vi "纳清蓝绿藻电极校准.vi"() -> ()   [LabVIEW 2016, in "斯坦道多参数.lvlib"]
uses:
  <vilib>/Utility/miscctls.llb/LVPointTypeDef.ctl
  <vilib>/Utility/miscctls.llb/LVPositionTypeDef.ctl
  <vilib>/Analysis/NI_AALBase.lvlib
panel:
  out "报警信息":string
  out "通讯状态":string
  out "温度校准参数":sgl
  out "第三点校准值":dbl
  out "标液3":sgl
  out "第二点校准值":dbl
  out "第一点校准值":dbl
  in  "校准停止":bool
  in  "校准启动":bool
  in  "校准模式":enum16{"两点校准", "单点校准", "三点校准"}(ring)=enum."单点校准"
  out "最小值":sgl format="%#.2f"
  out "最大值":sgl format="%#.2f"
  out "波形图表":u16(graph) caption="历史曲线"
  out "mean":dbl caption="均值" format="%#.2f"
  out "standard deviation":dbl caption="标准差" format="%#.2f"
  out "变异系数":dbl format="%#.6f"
  out "测量值":sgl
  out "提示":string
  out "标液2":sgl
  out "标液1":sgl
  out "原始光强数值":u16 caption="信号值"
  out "温度":dbl
  # "藻密度电极设定"
  # "℃"
  # "ug/L"
  # "℃"
  # "请选择校准模式:"
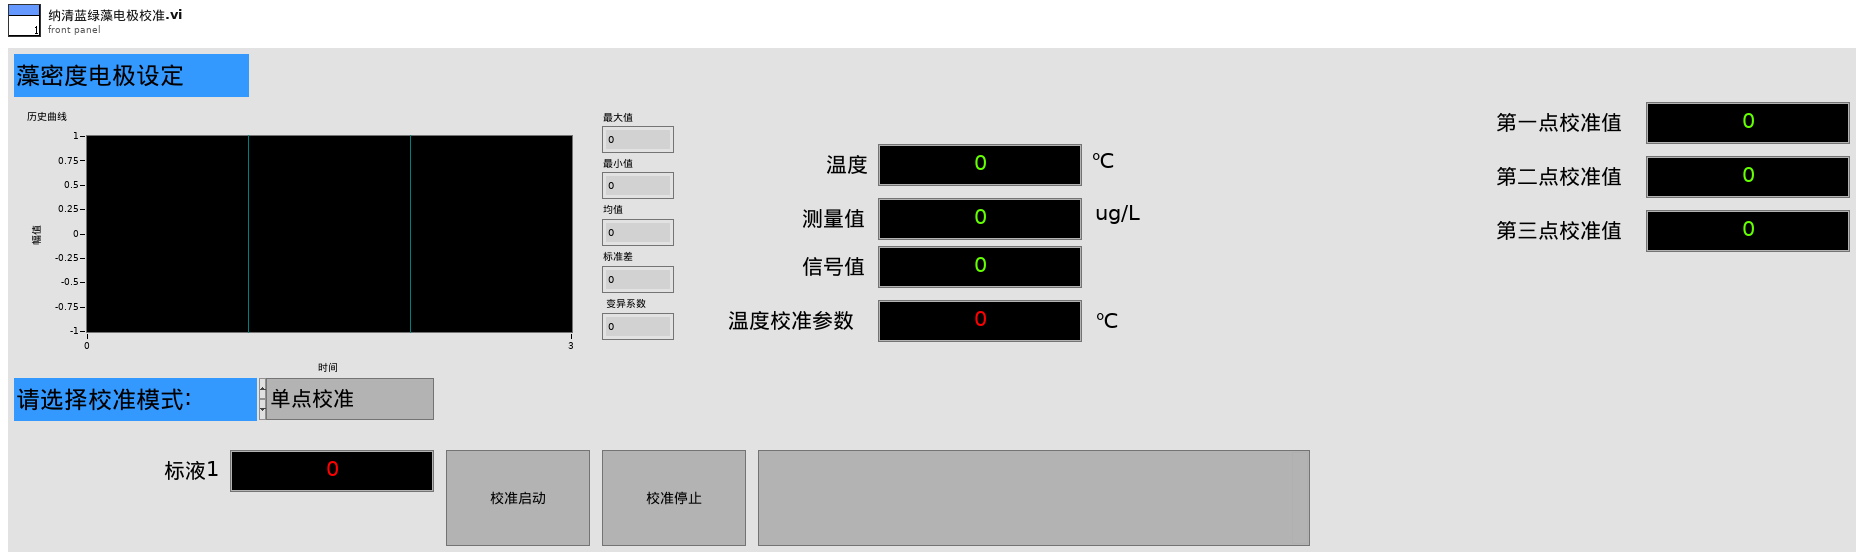
[diagram p1: front panel]
types:
  T1 = typedef "LVPointTypeDef.ctl" = cluster{"Horizontal":i16, "Vertical":i16}
  T2 = typedef "斯坦道多参数.lvlib/校准步骤.ctl" = enum16{"待机", "放置第一点标液", "第一点校准启动", "第一点校准写入", "第一点校准失败", "放置第二点标液", "第二点校准启动", "第二点校准写入", "第二点校准失败", "放置第三点标液", "第三点校准启动", "第三点校准写入", "第三点校准失败", "校准结果写入", "校准结束"}
  T3 = cluster{"报警码":u16, "蓝绿藻":sgl, "温度数据":sgl, "原始光强数值":u16, "0X0006_NC":u16, "平均次数":u16, "清扫模式":u16, "清扫次数":u16, "清扫间隔分钟":u16, "0X000B_NC":string, "产品名称":string, "序列号":string, "硬件版本":string, "软件版本":string, "通讯地址":u16, "波特率":u16, "设备类型":u16, "0X0026_NC":string, "0X0030_NC":u16, "第一点原始光强":u16, "第一点校准数据":sgl, "第二点原始光强":u16, "第二点校准数据":sgl, "第三点原始光强":u16, "第三点校准数据":sgl, "探头校准命令":u16, "温度校准参数":sgl, "温度校准命令":u16}
  T4 = typedef "LVPositionTypeDef.ctl" = cluster{"Left":i32, "Top":i32}
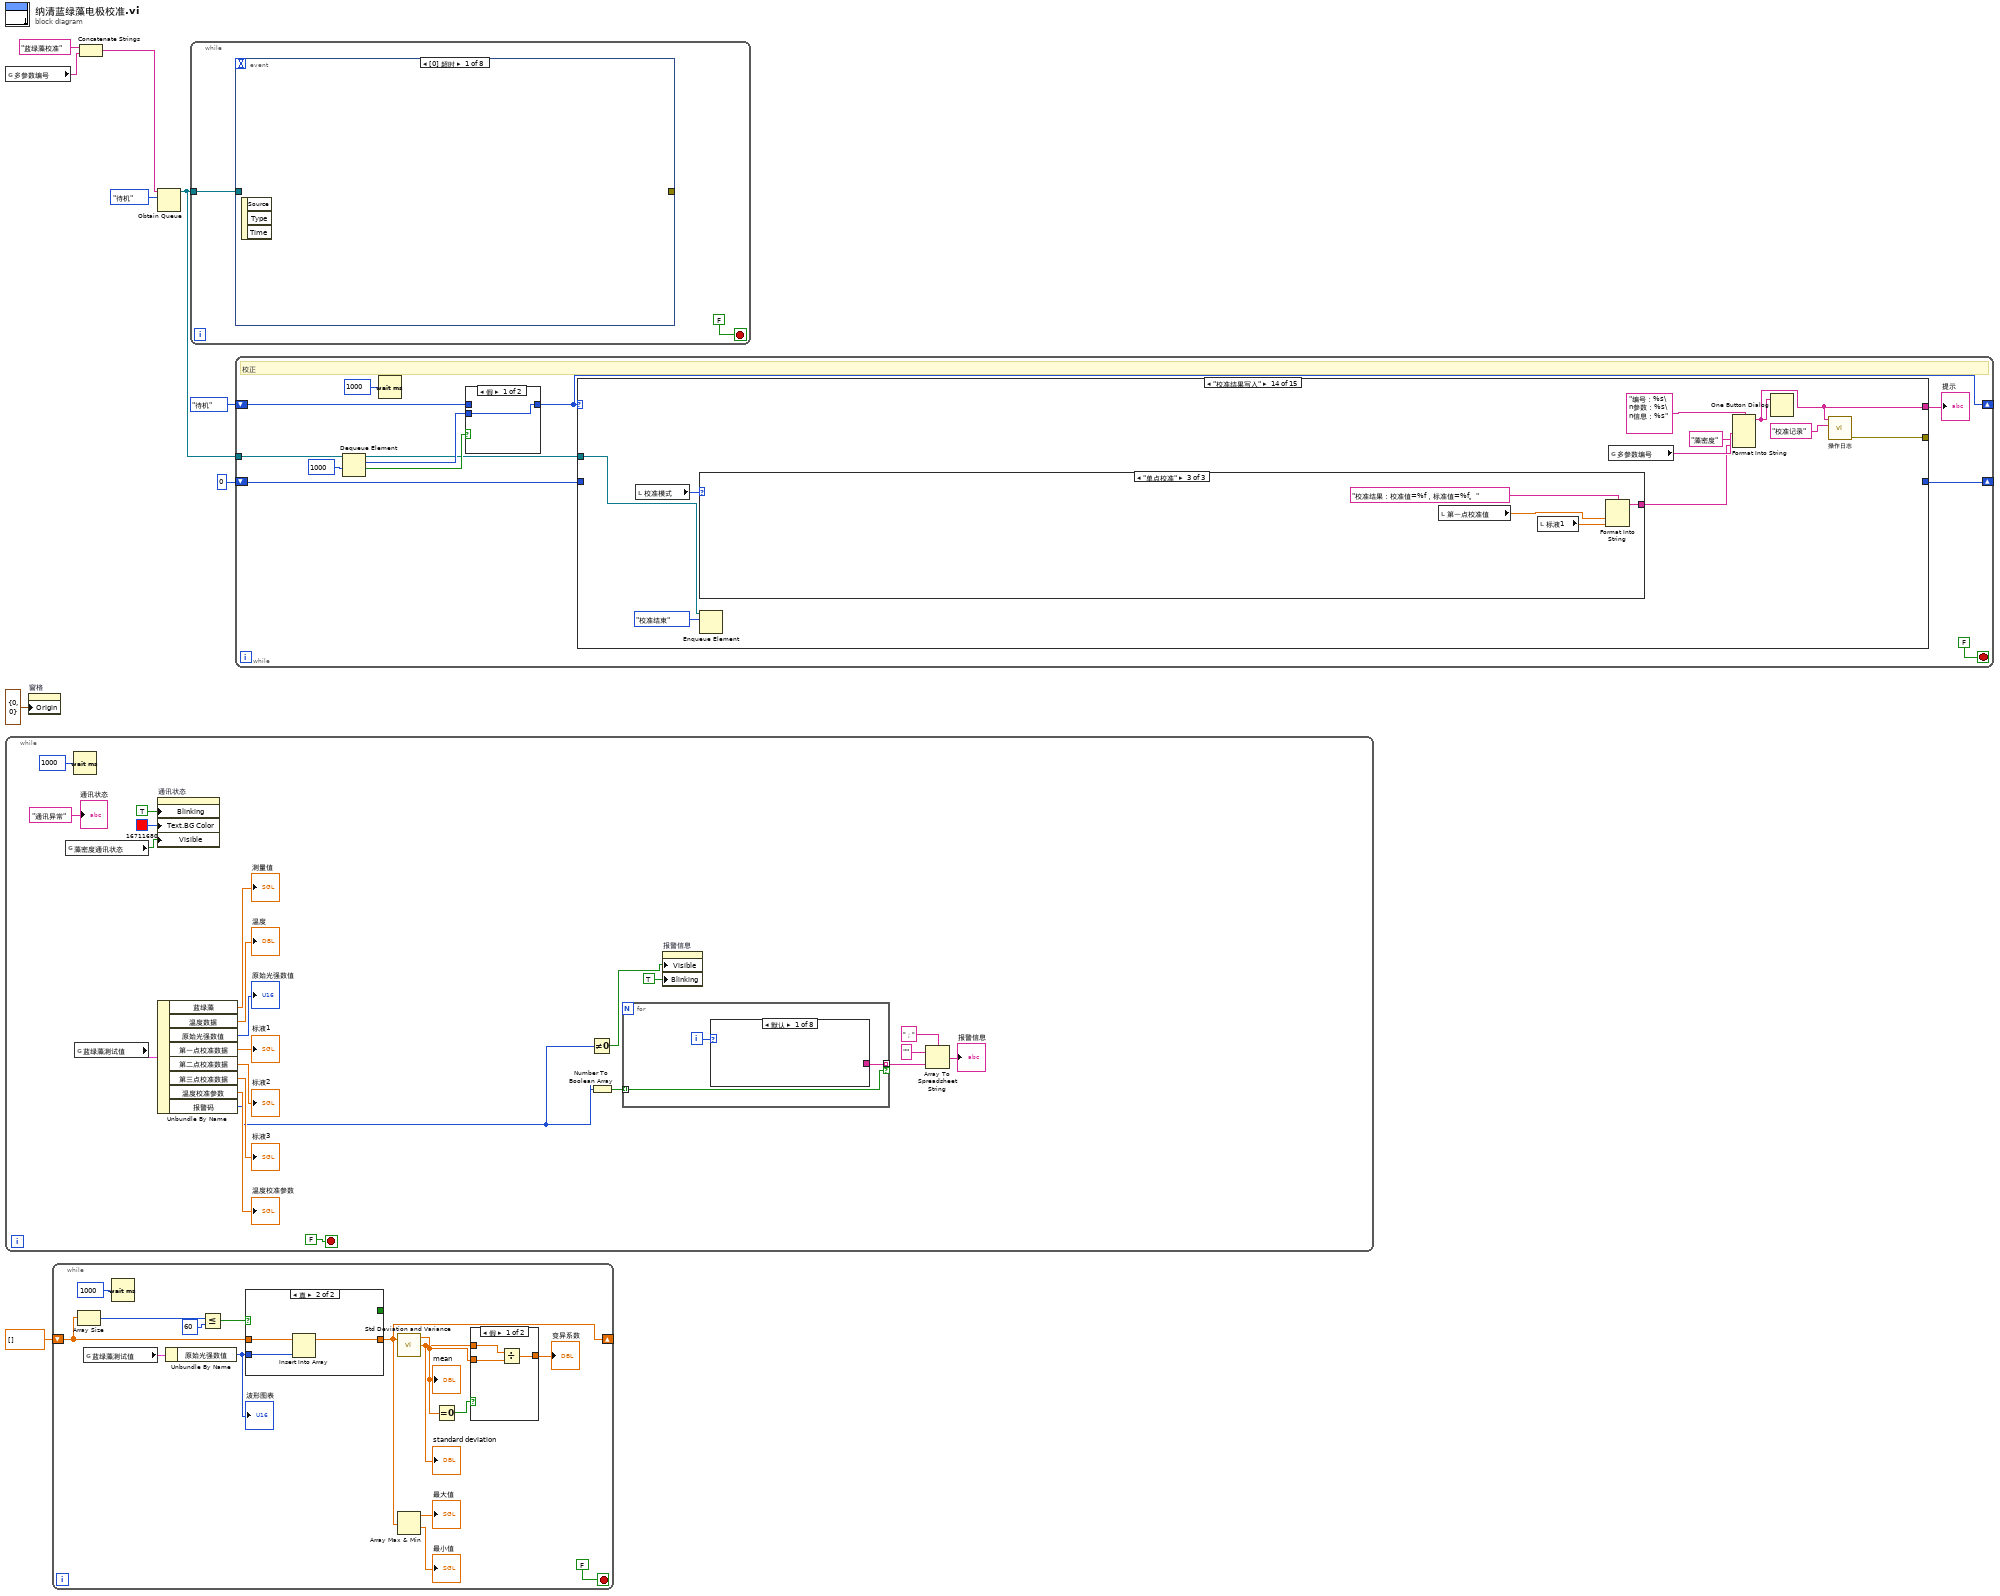
[diagram p0: block diagram]
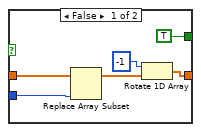
[diagram p3: hidden frame]
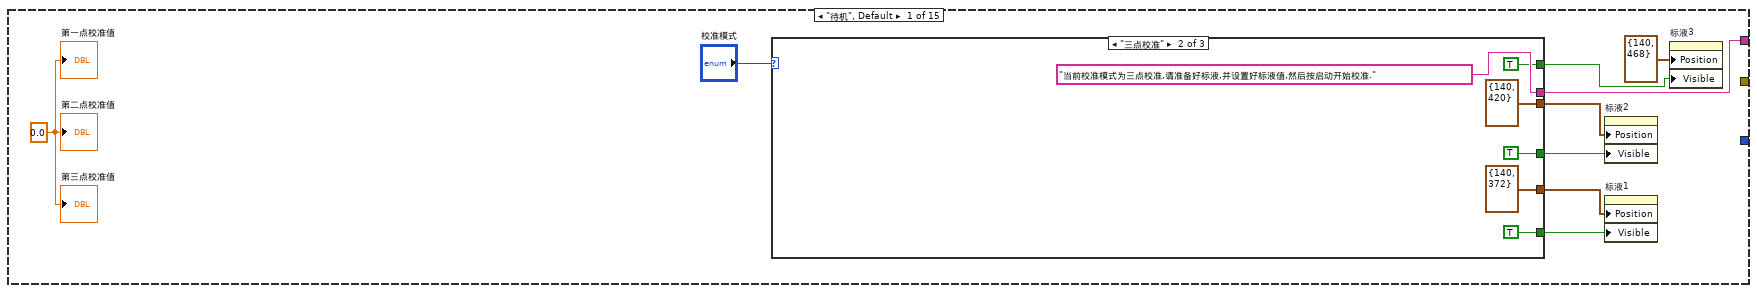
[diagram p5: hidden frame]
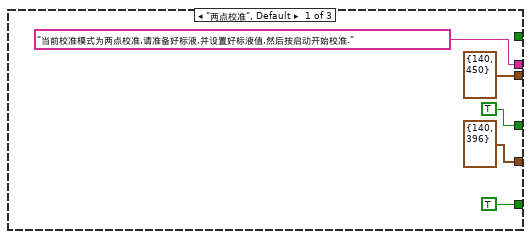
[diagram p6: hidden frame]
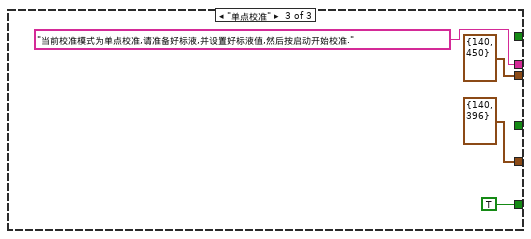
[diagram p7: hidden frame]
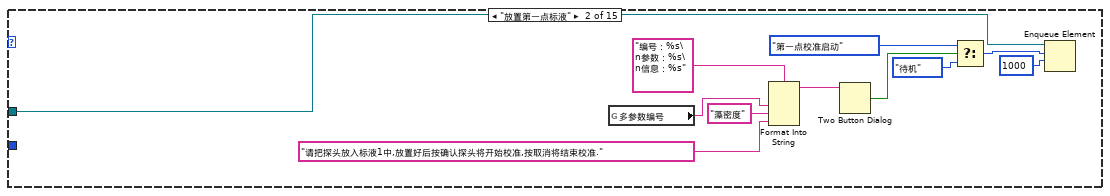
[diagram p8: hidden frame]
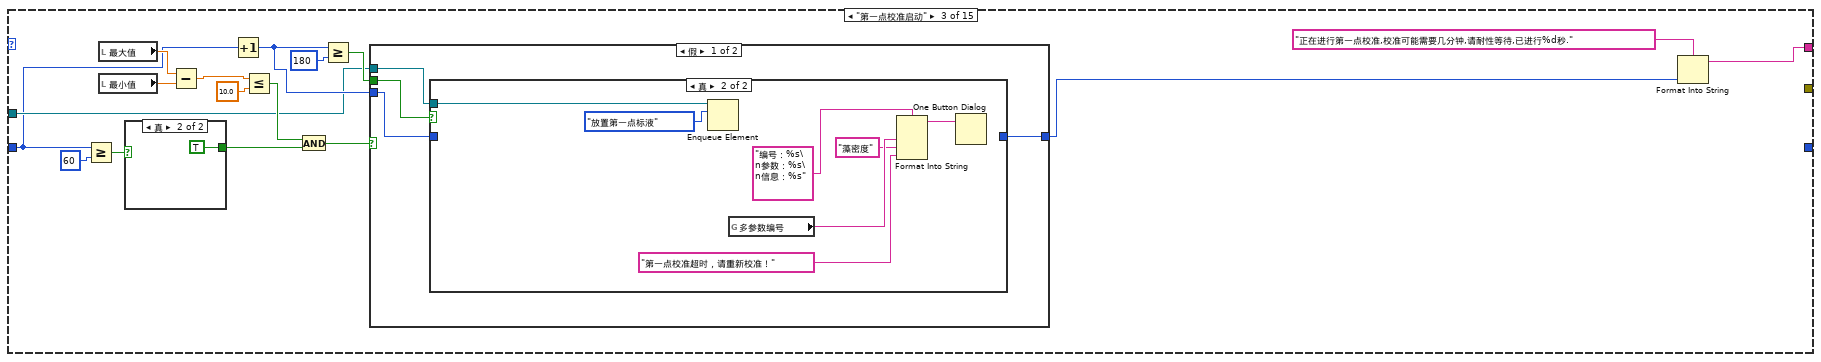
[diagram p9: hidden frame]
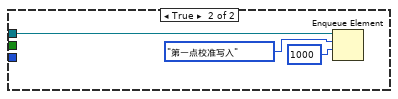
[diagram p11: hidden frame]
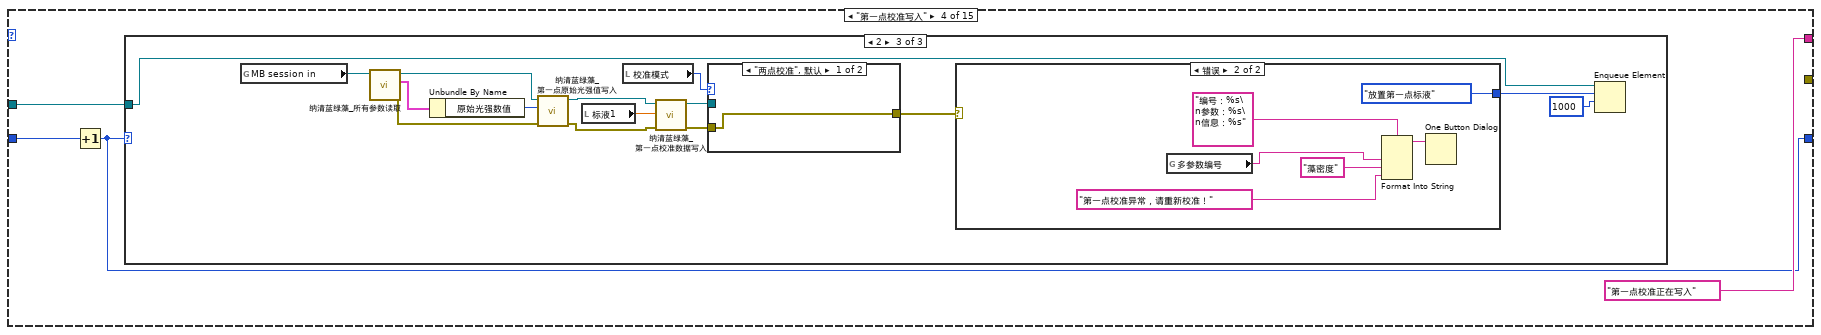
[diagram p13: hidden frame]
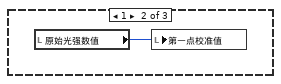
[diagram p15: hidden frame]
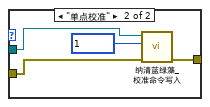
[diagram p16: hidden frame]
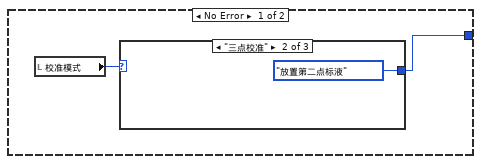
[diagram p17: hidden frame]
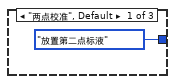
[diagram p18: hidden frame]
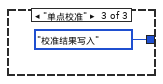
[diagram p19: hidden frame]
diagram:
  n1 = global read "多参数全局变量.vi" "多参数编号"() -> (w1:string)
  n2 = while {
    stop <- FALSE stop-if-true
    n3 = global read "多参数全局变量.vi" "藻密度通讯状态"() -> (w18:bool)
    n4 = Wait (ms)(milliseconds to wait=u32 1000 ("等待时间（毫秒）")) -> ()  [unwired: 1 out]
    n5 = global read "纳清过程全局变量.vi" "蓝绿藻测试值"() -> (w29:T3)
    n6 = property on="通讯状态" class="Str"("Blinking"=TRUE ("闪烁"), "Text.BG Color"=u32 16711680, "Visible"=w18) -> ()  [unwired: 2 in, 2 out]
    n7 = Unbundle By Name(w29) -> ("蓝绿藻"=→"测量值":sgl, "温度数据"=→"温度":sgl, "原始光强数值"=→"原始光强数值":u16, "第一点校准数据"=→"标液1":sgl, "第二点校准数据"=→"标液2":sgl, "第三点校准数据"=→"标液3":sgl, "温度校准参数"=→"温度校准参数":sgl, "报警码"=w10:u16)
    n8 = Not Equal To 0?(x=w10) -> (x != 0?=w12:bool)
    n9 = Number To Boolean Array(number=w10) -> (Boolean array=w17:bool[])
    n10 = for {
      tunnel: w17 -> [w32] mode=indexing
      tunnel: [w33] -> w16 mode=indexing if=w32
      i -> [w34]
      n11 = case shown="默认" w34 {
        tunnel: [_ "测量值超量程" "温度超量程" "光强信号超范围" "清扫中" "温度传感器故障" "电极故障" "内部电压基准故障"] -> w33
        frame Default {
        }
        frame 0 {
        }
        frame 2 {
        }
        frame 3 {
        }
        frame 4 {
        }
        frame 8 {
        }
        frame 9 {
        }
        frame 10 {
        }
      }
    }
    n12 = property on="报警信息" class="Str"("Visible"=w12, "Blinking"=TRUE ("闪烁")) -> ()  [unwired: 2 in, 2 out]
    n13 = Array To Spreadsheet String(delimiter (Tab)="；" ("分隔符(Tab)"), array=w16, 3:"" ("格式字符串")) -> (spreadsheet string=→"报警信息":string)
    "通讯状态" <- "通讯异常" ("当前串口")
  }
  n14 = property on="窗格" class="Pane"("Origin"=T1 {"Horizontal"=0, "Vertical"=0} ("原点")) -> ()  [unwired: 2 in, 2 out]
  n15 = while {
    shift-right: [w46] -> _
    shift-left: sgl[] [] -> [w52]
    stop <- FALSE stop-if-true
    n16 = Array Size(array=w52) -> (size(s)=w54:i32)
    n17 = global read "纳清过程全局变量.vi" "蓝绿藻测试值"() -> (w42:T3)
    n18 = Wait (ms)(milliseconds to wait=u32 1000 ("等待时间（毫秒）")) -> ()  [unwired: 1 out]
    n19 = Unbundle By Name(w42) -> ("原始光强数值"=w43:u16)
    "波形图表" <- w43
    n20 = Less Or Equal?(x=w54, y=60) -> (x <= y?=w53:bool)
    n21 = case shown="真" w53 {
      tunnel: w52 -> [w65 w68]
      tunnel: w43 -> [w63 w67]
      tunnel: [w61 w66] -> w46
      tunnel: [TRUE _] -> _
      frame False {
        n22 = Replace Array Subset(array=w65, new element=w63) -> (w64:sgl[])  [unwired: 1 in]
        n23 = Rotate 1D Array(1:w64, 2:-1 ("n")) -> (0:w61:sgl[])
      }
      frame True {
        n24 = Insert Into Array(array=w68, new element=w67) -> (w66:sgl[])  [unwired: 1 in]
      }
    }
    n25 = call <vilib>:"Std Deviation and Variance.vi"("X"=w46) -> ("mean"=w50:dbl, "standard deviation"=w49:dbl)  [unwired: 1 in, 1 out]
    "mean" <- w50
    "standard deviation" <- w49
    n26 = Array Max & Min(array=w46) -> (max value=→"最大值":sgl, min value=→"最小值":sgl)  [unwired: 2 out]
    n27 = Equal To 0?(x=w50) -> (x = 0?=w51:bool)
    n28 = case shown="假" w51 {
      tunnel: w49 -> [w59 _]
      tunnel: [w58 _] -> w48
      tunnel: w50 -> [w57 _]
      frame False {
        n29 = Divide(x=w59, y=w57) -> (x/y=w58:dbl)
      }
      frame True {
      }
    }
    "变异系数" <- w48
  }
  n30 = Concatenate Strings("蓝绿藻校准" ("名称（未命名）"), w1) -> (w2:string)
  n31 = Obtain Queue(name (unnamed)=w2, element data type=校准步骤."待机" ("枚举")) -> (queue out=w4:refnum<queue>)  [unwired: 3 in, 2 out]
  n32 = while {
    tunnel: w4 -> [w69]
    stop <- FALSE stop-if-true
    n33 = event shown="[0] 超时" {
      selector: _ -> [_ _ _ _ _ _ _ _]
      dyn-events: _ -> [_ _ _ _ _ _ _ _]
      timeout: _ -> [_ _ _ _ _ _ _ _]
      tunnel: [_ _ w76 w80 w83 w84 _ _] -> _
      tunnel: w69 -> [_ _ _ _ _ _ w91 w93]
      event Timeout {
        n34 = event-data() -> ()  [unwired: 1 in, 3 out]
      }
      event "标液1", "标液2", "标液3", "温度校准参数": Mouse Down {
        n35 = event-data() -> ("CtlRef"=w71:refnum<vi>)  [unwired: 1 in, 7 out]
        n36 = property class="DigNum (严格)"(reference=w71) -> (reference out=w72:refnum<vi>, "Value"=w73:sgl)  [unwired: 1 in, 1 out]
        n37 = call "数字键盘.vi"("OldNumber"=w73) -> ("NewNumber"=w74:dbl)  [unwired: 1 in]
        n38 = property class="DigNum (严格)"(reference=w72, "Val(Sgnl)"=w74) -> ()  [unwired: 1 in, 2 out]
      }
      event "标液1": Value Change {
        n39 = event-data() -> ("NewVal"=w75:sgl)  [unwired: 1 in, 5 out]
        n40 = global read "多参数全局变量.vi" "MB session in"() -> (w77:refnum<class "MB_Master.lvclass">)
        n41 = call "纳清蓝绿藻_第一点校准数据写入.vi"("数值"=w75, "MB session in"=w77) -> ("error out"=w76:errorcluster)  [unwired: 8 in, 1 out]
      }
      event "标液2": Value Change {
        n42 = event-data() -> ("NewVal"=w79:sgl)  [unwired: 1 in, 5 out]
        n43 = global read "多参数全局变量.vi" "MB session in"() -> (w78:refnum<class "MB_Master.lvclass">)
        n44 = call "纳清蓝绿藻_第二点校准数据写入.vi"("数值"=w79, "MB session in"=w78) -> ("error out"=w80:errorcluster)  [unwired: 8 in, 1 out]
      }
      event "标液3": Value Change {
        n45 = event-data() -> ("NewVal"=w81:sgl)  [unwired: 1 in, 5 out]
        n46 = global read "多参数全局变量.vi" "MB session in"() -> (w82:refnum<class "MB_Master.lvclass">)
        n47 = call "纳清蓝绿藻_第三点校准数据写入.vi"("数值"=w81, "MB session in"=w82) -> ("error out"=w83:errorcluster)  [unwired: 8 in, 1 out]
      }
      event "温度校准参数": Value Change {
        n48 = event-data() -> ("NewVal"=w89:sgl)  [unwired: 1 in, 5 out]
        n49 = global read "多参数全局变量.vi" "MB session in"() -> (w88:refnum<class "MB_Master.lvclass">)
        n50 = call "纳清蓝绿藻_温度校准参数写入.vi"("数值"=w89, "MB session in"=w88) -> ("error out"=w90:errorcluster, "MB session out"=w87:refnum<class "MB_Master.lvclass">)  [unwired: 8 in]
        n51 = call "纳清蓝绿藻_温度校准命令写入.vi"("error in (no error)"=w90, "数值"=u16 1 ("starting address"), "MB session in"=w87) -> ("error out"=w85:errorcluster)  [unwired: 7 in, 1 out]
        n52 = call <vilib>:"Simple Error Handler.vi"("error in (no error)"=w85) -> ("error out"=w84:errorcluster)  [unwired: 4 in, 4 out]
      }
      event "校准启动": Value Change {
        n53 = event-data() -> ()  [unwired: 1 in, 6 out]
        n54 = Enqueue Element(queue=w91, element=校准步骤."放置第一点标液" ("元素")) -> ()  [unwired: 2 in, 3 out]
      }
      event "校准停止": Value Change {
        n55 = event-data() -> ()  [unwired: 1 in, 6 out]
        n56 = Flush Queue(queue=w93) -> (queue out=w94:refnum<queue>)  [unwired: 1 in, 2 out]
        n57 = Enqueue Element(queue=w94, element=校准步骤."待机" ("元素"), timeout in ms (-1)=1000 ("超时毫秒(-1)")) -> ()  [unwired: 1 in, 3 out]
      }
    }
  }
  n58 = while "While循环" {
    shift-right: [w98] -> _
    shift-left: 校准步骤."待机" ("枚举") -> [w100]
    shift-right: [w97] -> _
    shift-left: 0 -> [w106]
    tunnel: w4 -> [w101]
    stop <- FALSE stop-if-true
    # "校正"
    n59 = Dequeue Element(queue=w101, timeout in ms (-1)=1000 ("超时毫秒(-1)")) -> (queue out=w99:refnum<queue>, element=w102:T2, timed out?=w103:bool)  [unwired: 1 in, 1 out]
    n60 = Wait (ms)(milliseconds to wait=u32 1000 ("等待时间（毫秒）")) -> ()  [unwired: 1 out]
    n61 = case shown="假" w103 {
      tunnel: w102 -> [w109 _]
      tunnel: [w109 w110] -> w98
      tunnel: w100 -> [_ w110]
      frame False {
      }
      frame True {
      }
    }
    n62 = case shown="\"校准结果写入\"" w98 {
      tunnel: [w118 _ w146 "第一点校准正在写入" ("提示") _ _ w228 "第二点校准正在写入" ("提示") "第二点校准失败" ("提示") _ "第三点校准正在写入" ("提示") w340 "第三点校准失败" ("提示") w373 w400] -> w105
      tunnel: w106 -> [_ _ w148 w181 _ _ w229 w261 _ _ w309 w341 _ _ _]
      tunnel: [_ _ _ w179 _ _ w227 w259 _ _ w307 w339 _ _ _] -> w97
      tunnel: w99 -> [_ w141 w149 w180 _ w220 w230 w260 _ w301 w308 w342 _ w380 _]
      tunnel: [_ _ _ _ _ _ _ _ _ _ _ _ _ w378 _] -> _
      frame "待机", Default {
        w111 = 0.0 ("第一点校准值")
        n63 = case shown="\"三点校准\"" "校准模式" {
          tunnel: ["当前校准模式为两点校准,请准备好标液,并设置好标液值,然后按启动开始校准." ("提示") "当前校准模式为三点校准,请准备好标液,并设置好标液值,然后按启动开始校准." ("提示") "当前校准模式为单点校准,请准备好标液,并设置好标液值,然后按启动开始校准." ("提示")] -> w118
          tunnel: [TRUE ("可见") TRUE ("可见") _] -> w114
          tunnel: [T4 {"Left"=140, "Top"=396} ("位置") T4 {"Left"=140, "Top"=372} ("位置") T4 {"Left"=140, "Top"=396} ("位置")] -> w117
          tunnel: [T4 {"Left"=140, "Top"=450} ("位置 2") T4 {"Left"=140, "Top"=420} ("位置 2") T4 {"Left"=140, "Top"=450} ("位置 2")] -> w116
          tunnel: [_ TRUE ("可见") _] -> w113
          tunnel: [TRUE ("可见") TRUE ("可见") TRUE ("可见")] -> w112
          frame "两点校准", Default {
          }
          frame "三点校准" {
          }
          frame "单点校准" {
          }
        }
        n64 = property on="标液2" class="DigNum (严格)"("Position"=w116, "Visible"=w114) -> ()  [unwired: 2 in, 2 out]
        n65 = property on="标液1" class="DigNum (严格)"("Position"=w117, "Visible"=w112) -> ()  [unwired: 2 in, 2 out]
        n66 = property on="标液3" class="DigNum (严格)"("Position"=T4 {"Left"=140, "Top"=468} ("位置 3"), "Visible"=w113) -> ()  [unwired: 2 in, 2 out]
        "第一点校准值" <- w111
        "第二点校准值" <- w111
        "第三点校准值" <- w111
      }
      frame "放置第一点标液" {
        n67 = global read "多参数全局变量.vi" "多参数编号"() -> (w139:string)
        n68 = Format Into String(format string="编号：%s\n参数：%s\n信息：%s" ("格式字符串"), w139, "藻密度" ("输入 2"), "请把探头放入标液1中,放置好后按确认探头将开始校准,按取消将结束校准." ("消息")) -> (resulting string=w137:string)  [unwired: 2 in, 1 out]
        n69 = Two Button Dialog(message=w137) -> (T button?=w135:bool)  [unwired: 2 in]
        n70 = Select(t=校准步骤."第一点校准启动" ("元素"), s=w135, f=校准步骤."待机" ("元素")) -> (s? t:f=w142:T2)
        n71 = Enqueue Element(queue=w141, element=w142, timeout in ms (-1)=1000 ("超时毫秒(-1)")) -> ()  [unwired: 1 in, 3 out]
      }
      frame "第一点校准启动" {
        n72 = Greater Or Equal?(x=w148, y=60) -> (x >= y?=w155:bool)
        n73 = local read "最大值"() -> (w158:sgl)
        n74 = local read "最小值"() -> (w157:sgl)
        n75 = case shown="真" w155 {
          tunnel: [_ TRUE] -> w156
          frame False {
          }
          frame True {
          }
        }
        n76 = Subtract(x=w158, y=w157) -> (x-y=w159:sgl)
        n77 = Increment(x=w148) -> (x+1=w162:i32)
        n78 = Less Or Equal?(x=w159, y=10.0) -> (x <= y?=w152:bool)
        n79 = And(x=w152, y=w156) -> (x .and. y?=w160:bool)
        n80 = Greater Or Equal?(x=w162, y=180) -> (x >= y?=w161:bool)
        n81 = case shown="假" w160 {
          tunnel: w149 -> [w165 w177]
          tunnel: w161 -> [w166 _]
          tunnel: w162 -> [w164 _]
          tunnel: [w163 _] -> w147
          frame False {
            n82 = case shown="真" w166 {
              tunnel: w165 -> [_ w174]
              tunnel: w164 -> [w167 _]
              tunnel: [w167 _] -> w163
              frame False {
              }
              frame True {
                n83 = Enqueue Element(queue=w174, element=校准步骤."放置第一点标液" ("元素")) -> ()  [unwired: 2 in, 3 out]
                n84 = global read "多参数全局变量.vi" "多参数编号"() -> (w171:string)
                n85 = Format Into String(format string="编号：%s\n参数：%s\n信息：%s" ("格式字符串"), w171, "藻密度" ("输入 2"), "第一点校准超时，请重新校准！" ("error source (\" \")")) -> (resulting string=w168:string)  [unwired: 2 in, 1 out]
                n86 = One Button Dialog(message=w168) -> ()  [unwired: 1 in, 1 out]
              }
            }
          }
          frame True {
            n87 = Enqueue Element(queue=w177, element=校准步骤."第一点校准写入" ("元素"), timeout in ms (-1)=1000 ("超时毫秒(-1)")) -> ()  [unwired: 1 in, 3 out]
          }
        }
        n88 = Format Into String(format string="正在进行第一点校准,校准可能需要几分钟,请耐性等待,已进行%d秒." ("格式字符串"), w147) -> (resulting string=w146:string)  [unwired: 2 in, 1 out]
      }
      frame "第一点校准写入" {
        n89 = Increment(x=w181) -> (x+1=w179:i32)
        n90 = case shown="2" w179 {
          tunnel: w180 -> [_ _ w198]
          frame 0, Default {
          }
          frame 1 {
            n91 = local read "原始光强数值"() -> (w183:u16)
            n92 = local write "第一点校准值"(w183) -> ()
          }
          frame 2 {
            n93 = global read "多参数全局变量.vi" "MB session in"() -> (w194:refnum<class "MB_Master.lvclass">)
            n94 = call "纳清蓝绿藻_所有参数读取.vi"("MB session in"=w194) -> ("error out"=w196:errorcluster, "输出值"=w193:T3, "MB session out"=w195:refnum<class "MB_Master.lvclass">)  [unwired: 8 in]
            n95 = Unbundle By Name(w193) -> ("原始光强数值"=w192:u16)
            n96 = call "纳清蓝绿藻_第一点原始光强值写入.vi"("error in (no error)"=w196, "数值"=w192, "MB session in"=w195) -> ("error out"=w191:errorcluster, "MB session out"=w190:refnum<class "MB_Master.lvclass">)  [unwired: 7 in]
            n97 = local read "标液1"() -> (w187:sgl)
            n98 = local read "校准模式"() -> (w184:enum16{"两点校准", "单点校准", "三点校准"})
            n99 = call "纳清蓝绿藻_第一点校准数据写入.vi"("error in (no error)"=w191, "数值"=w187, "MB session in"=w190) -> ("error out"=w189:errorcluster, "MB session out"=w188:refnum<class "MB_Master.lvclass">)  [unwired: 7 in]
            n100 = case shown="\"两点校准\", 默认" w184 {
              tunnel: w189 -> [w199 w203]
              tunnel: w188 -> [_ w202]
              tunnel: [w199 w200] -> w186
              frame "两点校准", Default {
              }
              frame "单点校准" {
                n101 = call "纳清蓝绿藻_校准命令写入.vi"("error in (no error)"=w203, "数值"=u16 1 ("starting address"), "MB session in"=w202) -> ("error out"=w200:errorcluster)  [unwired: 7 in, 1 out]
              }
            }
            n102 = case shown="错误" w186 {
              tunnel: [w204 校准步骤."放置第一点标液" ("元素")] -> w185
              frame No Error {
                n103 = local read "校准模式"() -> (w205:enum16{"两点校准", "单点校准", "三点校准"})
                n104 = case shown="\"三点校准\"" w205 {
                  tunnel: [校准步骤."放置第二点标液" ("元素") 校准步骤."放置第二点标液" ("元素") 校准步骤."校准结果写入" ("元素")] -> w204
                  frame "两点校准", Default {
                  }
                  frame "三点校准" {
                  }
                  frame "单点校准" {
                  }
                }
              }
              frame Error {
                n105 = global read "多参数全局变量.vi" "多参数编号"() -> (w213:string)
                n106 = Format Into String(format string="编号：%s\n参数：%s\n信息：%s" ("格式字符串"), w213, "藻密度" ("输入 2"), "第一点校准异常，请重新校准！" ("error source (\" \")")) -> (resulting string=w210:string)  [unwired: 2 in, 1 out]
                n107 = One Button Dialog(message=w210) -> ()  [unwired: 1 in, 1 out]
              }
            }
            n108 = Enqueue Element(queue=w198, element=w185, timeout in ms (-1)=1000 ("超时毫秒(-1)")) -> ()  [unwired: 1 in, 3 out]
          }
        }
      }
      frame "第一点校准失败" {
      }
      frame "放置第二点标液" {
        n109 = global read "多参数全局变量.vi" "多参数编号"() -> (w218:string)
        n110 = Format Into String(format string="编号：%s\n参数：%s\n信息：%s" ("格式字符串"), w218, "藻密度" ("输入 2"), "请把探头放入标液2中,放置好后按确认将继续校准,按取消将结束校准." ("消息")) -> (resulting string=w216:string)  [unwired: 2 in, 1 out]
        n111 = Two Button Dialog(message=w216) -> (T button?=w224:bool)  [unwired: 2 in]
        n112 = Select(t=校准步骤."第二点校准启动" ("元素"), s=w224, f=校准步骤."待机" ("元素")) -> (s? t:f=w221:T2)
        n113 = Enqueue Element(queue=w220, element=w221, timeout in ms (-1)=1000 ("超时毫秒(-1)")) -> ()  [unwired: 1 in, 3 out]
      }
      frame "第二点校准启动" {
        n114 = Greater Or Equal?(x=w229, y=60) -> (x >= y?=w235:bool)
        n115 = local read "最大值"() -> (w238:sgl)
        n116 = local read "最小值"() -> (w237:sgl)
        n117 = case shown="真" w235 {
          tunnel: [_ TRUE] -> w236
          frame False {
          }
          frame True {
          }
        }
        n118 = Subtract(x=w238, y=w237) -> (x-y=w239:sgl)
        n119 = Increment(x=w229) -> (x+1=w242:i32)
        n120 = Less Or Equal?(x=w239, y=10.0) -> (x <= y?=w232:bool)
        n121 = And(x=w232, y=w236) -> (x .and. y?=w240:bool)
        n122 = Greater Or Equal?(x=w242, y=180) -> (x >= y?=w241:bool)
        n123 = case shown="假" w240 {
          tunnel: w230 -> [w245 w257]
          tunnel: w241 -> [w246 _]
          tunnel: w242 -> [w244 _]
          tunnel: [w243 _] -> w227
          frame False {
            n124 = case shown="真" w246 {
              tunnel: w245 -> [_ w254]
              tunnel: w244 -> [w247 _]
              tunnel: [w247 _] -> w243
              frame False {
              }
              frame True {
                n125 = Enqueue Element(queue=w254, element=校准步骤."放置第二点标液" ("元素")) -> ()  [unwired: 2 in, 3 out]
                n126 = global read "多参数全局变量.vi" "多参数编号"() -> (w251:string)
                n127 = Format Into String(format string="编号：%s\n参数：%s\n信息：%s" ("格式字符串"), w251, "藻密度" ("输入 2"), "第二点校准超时，请重新校准！" ("消息")) -> (resulting string=w249:string)  [unwired: 2 in, 1 out]
                n128 = One Button Dialog(message=w249) -> ()  [unwired: 1 in, 1 out]
              }
            }
          }
          frame True {
            n129 = Enqueue Element(queue=w257, element=校准步骤."第二点校准写入" ("元素"), timeout in ms (-1)=1000 ("超时毫秒(-1)")) -> ()  [unwired: 1 in, 3 out]
          }
        }
        n130 = Format Into String(format string="正在进行第二点校准,校准可能需要几分钟,请耐性等待,已进行%d秒." ("格式字符串"), w227) -> (resulting string=w228:string)  [unwired: 2 in, 1 out]
      }
      frame "第二点校准写入" {
        n131 = Increment(x=w261) -> (x+1=w259:i32)
        n132 = case shown="2" w259 {
          tunnel: w260 -> [_ _ w278]
          frame 0, Default {
          }
          frame 1 {
            n133 = local read "原始光强数值"() -> (w263:u16)
            n134 = local write "第二点校准值"(w263) -> ()
          }
          frame 2 {
            n135 = global read "多参数全局变量.vi" "MB session in"() -> (w274:refnum<class "MB_Master.lvclass">)
            n136 = call "纳清蓝绿藻_所有参数读取.vi"("MB session in"=w274) -> ("error out"=w276:errorcluster, "输出值"=w273:T3, "MB session out"=w275:refnum<class "MB_Master.lvclass">)  [unwired: 8 in]
            n137 = Unbundle By Name(w273) -> ("原始光强数值"=w272:u16)
            n138 = call "纳清蓝绿藻_第二点原始光强值写入.vi"("error in (no error)"=w276, "数值"=w272, "MB session in"=w275) -> ("error out"=w271:errorcluster, "MB session out"=w270:refnum<class "MB_Master.lvclass">)  [unwired: 7 in]
            n139 = local read "标液2"() -> (w267:sgl)
            n140 = local read "校准模式"() -> (w264:enum16{"两点校准", "单点校准", "三点校准"})
            n141 = call "纳清蓝绿藻_第二点校准数据写入.vi"("error in (no error)"=w271, "数值"=w267, "MB session in"=w270) -> ("error out"=w269:errorcluster, "MB session out"=w268:refnum<class "MB_Master.lvclass">)  [unwired: 7 in]
            n142 = case shown="\"两点校准\"" w264 {
              tunnel: w269 -> [w282 w283]
              tunnel: w268 -> [w281 _]
              tunnel: [w279 w283] -> w266
              frame "两点校准" {
                n143 = call "纳清蓝绿藻_校准命令写入.vi"("error in (no error)"=w282, "数值"=u16 2 ("starting address"), "MB session in"=w281) -> ("error out"=w279:errorcluster)  [unwired: 7 in, 1 out]
              }
              frame "单点校准", Default {
              }
            }
            n144 = case shown="错误" w266 {
              tunnel: [w284 校准步骤."放置第二点标液" ("元素")] -> w265
              frame No Error {
                n145 = local read "校准模式"() -> (w285:enum16{"两点校准", "单点校准", "三点校准"})
                n146 = case shown="\"单点校准\"" w285 {
                  tunnel: [校准步骤."校准结果写入" ("元素") 校准步骤."放置第三点标液" ("元素") 校准步骤."校准结果写入" ("元素")] -> w284
                  frame "两点校准", Default {
                  }
                  frame "三点校准" {
                  }
                  frame "单点校准" {
                  }
                }
              }
              frame Error {
                n147 = global read "多参数全局变量.vi" "多参数编号"() -> (w293:string)
                n148 = Format Into String(format string="编号：%s\n参数：%s\n信息：%s" ("格式字符串"), w293, "藻密度" ("输入 2"), "第二点校准异常，请重新校准！" ("error source (\" \")")) -> (resulting string=w290:string)  [unwired: 2 in, 1 out]
                n149 = One Button Dialog(message=w290) -> ()  [unwired: 1 in, 1 out]
              }
            }
            n150 = Enqueue Element(queue=w278, element=w265, timeout in ms (-1)=1000 ("超时毫秒(-1)")) -> ()  [unwired: 1 in, 3 out]
          }
        }
      }
      frame "第二点校准失败" {
      }
      frame "放置第三点标液" {
        n151 = global read "多参数全局变量.vi" "多参数编号"() -> (w299:string)
        n152 = Format Into String(format string="编号：%s\n参数：%s\n信息：%s" ("格式字符串"), w299, "藻密度" ("输入 2"), "请把探头放入标液3中,放置好后按确认将继续校准,按取消将结束校准." ("消息")) -> (resulting string=w297:string)  [unwired: 2 in, 1 out]
        n153 = Two Button Dialog(message=w297) -> (T button?=w305:bool)  [unwired: 2 in]
        n154 = Select(t=校准步骤."第三点校准启动" ("元素"), s=w305, f=校准步骤."待机" ("元素")) -> (s? t:f=w302:T2)
        n155 = Enqueue Element(queue=w301, element=w302, timeout in ms (-1)=1000 ("超时毫秒(-1)")) -> ()  [unwired: 1 in, 3 out]
      }
      frame "第三点校准写入" {
        n156 = Increment(x=w309) -> (x+1=w307:i32)
        n157 = case shown="2" w307 {
          tunnel: w308 -> [_ _ w313]
          frame 0, Default {
          }
          frame 1 {
            n158 = local read "原始光强数值"() -> (w311:u16)
            n159 = local write "第二点校准值"(w311) -> ()
          }
          frame 2 {
            n160 = global read "多参数全局变量.vi" "MB session in"() -> (w324:refnum<class "MB_Master.lvclass">)
            n161 = call "纳清蓝绿藻_所有参数读取.vi"("MB session in"=w324) -> ("error out"=w326:errorcluster, "输出值"=w323:T3, "MB session out"=w325:refnum<class "MB_Master.lvclass">)  [unwired: 8 in]
            n162 = Unbundle By Name(w323) -> ("原始光强数值"=w322:u16)
            n163 = call "纳清蓝绿藻_第三点原始光强值写入.vi"("error in (no error)"=w326, "数值"=w322, "MB session in"=w325) -> ("error out"=w321:errorcluster, "MB session out"=w320:refnum<class "MB_Master.lvclass">)  [unwired: 7 in]
            n164 = local read "标液3"() -> (w316:sgl)
            n165 = call "纳清蓝绿藻_第三点校准数据写入.vi"("error in (no error)"=w321, "数值"=w316, "MB session in"=w320) -> ("error out"=w319:errorcluster, "MB session out"=w318:refnum<class "MB_Master.lvclass">)  [unwired: 7 in]
            n166 = call "纳清蓝绿藻_校准命令写入.vi"("error in (no error)"=w319, "数值"=u16 3 ("starting address"), "MB session in"=w318) -> ("error out"=w315:errorcluster)  [unwired: 7 in, 1 out]
            n167 = case shown="错误" w315 {
              tunnel: [w327 校准步骤."放置第三点标液" ("元素")] -> w312
              frame No Error {
                n168 = local read "校准模式"() -> (w328:enum16{"两点校准", "单点校准", "三点校准"})
                n169 = case shown="\"三点校准\"" w328 {
                  tunnel: [校准步骤."放置第二点标液" ("元素") 校准步骤."校准结果写入" ("元素") 校准步骤."校准结果写入" ("元素")] -> w327
                  frame "两点校准", Default {
                  }
                  frame "三点校准" {
                  }
                  frame "单点校准" {
                  }
                }
              }
              frame Error {
                n170 = global read "多参数全局变量.vi" "多参数编号"() -> (w336:string)
                n171 = Format Into String(format string="编号：%s\n参数：%s\n信息：%s" ("格式字符串"), w336, "藻密度" ("输入 2"), "第三点校准异常，请重新校准！" ("error source (\" \")")) -> (resulting string=w333:string)  [unwired: 2 in, 1 out]
                n172 = One Button Dialog(message=w333) -> ()  [unwired: 1 in, 1 out]
              }
            }
            n173 = Enqueue Element(queue=w313, element=w312, timeout in ms (-1)=1000 ("超时毫秒(-1)")) -> ()  [unwired: 1 in, 3 out]
          }
        }
      }
      frame "第三点校准启动" {
        n174 = Greater Or Equal?(x=w341, y=60) -> (x >= y?=w347:bool)
        n175 = local read "最大值"() -> (w350:sgl)
        n176 = local read "最小值"() -> (w349:sgl)
        n177 = case shown="真" w347 {
          tunnel: [_ TRUE] -> w348
          frame False {
          }
          frame True {
          }
        }
        n178 = Subtract(x=w350, y=w349) -> (x-y=w351:sgl)
        n179 = Increment(x=w341) -> (x+1=w354:i32)
        n180 = Less Or Equal?(x=w351, y=10.0) -> (x <= y?=w344:bool)
        n181 = And(x=w344, y=w348) -> (x .and. y?=w352:bool)
        n182 = Greater Or Equal?(x=w354, y=180) -> (x >= y?=w353:bool)
        n183 = case shown="假" w352 {
          tunnel: w342 -> [w357 w369]
          tunnel: w353 -> [w358 _]
          tunnel: w354 -> [w356 _]
          tunnel: [w355 _] -> w339
          frame False {
            n184 = case shown="真" w358 {
              tunnel: w357 -> [_ w366]
              tunnel: w356 -> [w359 _]
              tunnel: [w359 _] -> w355
              frame False {
              }
              frame True {
                n185 = Enqueue Element(queue=w366, element=校准步骤."放置第三点标液" ("元素")) -> ()  [unwired: 2 in, 3 out]
                n186 = global read "多参数全局变量.vi" "多参数编号"() -> (w363:string)
                n187 = Format Into String(format string="编号：%s\n参数：%s\n信息：%s" ("格式字符串"), w363, "藻密度" ("输入 2"), "第三点校准异常，请重新校准！" ("error source (\" \")")) -> (resulting string=w360:string)  [unwired: 2 in, 1 out]
                n188 = One Button Dialog(message=w360) -> ()  [unwired: 1 in, 1 out]
              }
            }
          }
          frame True {
            n189 = Enqueue Element(queue=w369, element=校准步骤."第三点校准写入" ("元素"), timeout in ms (-1)=1000 ("超时毫秒(-1)")) -> ()  [unwired: 1 in, 3 out]
          }
        }
        n190 = Format Into String(format string="正在进行第三点校准,校准可能需要几分钟,请耐性等待,已进行%d秒." ("格式字符串"), w339) -> (resulting string=w340:string)  [unwired: 2 in, 1 out]
      }
      frame "第三点校准失败" {
      }
      frame "校准结果写入" {
        n191 = local read "校准模式"() -> (w379:enum16{"两点校准", "单点校准", "三点校准"})
        n192 = case shown="\"单点校准\"" w379 {
          tunnel: [w384 w392 w399] -> w374
          frame "两点校准", Default {
            n193 = local read "第一点校准值"() -> (w387:dbl)
            n194 = local read "第二点校准值"() -> (w383:dbl)
            n195 = local read "标液1"() -> (w385:sgl)
            n196 = local read "标液2"() -> (w382:sgl)
            n197 = Format Into String(format string="校准结果：第一点校准值=%f，第一点标准值=%f,第二点校准值=%f，第二点标准值=%f." ("提示"), w387, w385, w383, w382) -> (resulting string=w384:string)  [unwired: 2 in, 1 out]
          }
          frame "三点校准" {
            n198 = local read "第一点校准值"() -> (w395:dbl)
            n199 = local read "第二点校准值"() -> (w391:dbl)
            n200 = local read "第三点校准值"() -> (w389:dbl)
            n201 = local read "标液1"() -> (w393:sgl)
            n202 = local read "标液2"() -> (w390:sgl)
            n203 = local read "标液3"() -> (w388:sgl)
            n204 = Format Into String(format string="校准结果：第一点校准值=%f，第一点标准值=%f,第二点校准值=%f，第二点标准值=%f,第三点校准值=%f，第三点标准值=%f." ("提示"), w395, w393, w391, w390, w389, w388) -> (resulting string=w392:string)  [unwired: 2 in, 1 out]
          }
          frame "单点校准" {
            n205 = local read "第一点校准值"() -> (w398:dbl)
            n206 = local read "标液1"() -> (w396:sgl)
            n207 = Format Into String(format string="校准结果：校准值=%f，标准值=%f。" ("提示"), w398, w396) -> (resulting string=w399:string)  [unwired: 2 in, 1 out]
          }
        }
        n208 = Enqueue Element(queue=w380, element=校准步骤."校准结束" ("元素")) -> ()  [unwired: 2 in, 3 out]
        n209 = global read "多参数全局变量.vi" "多参数编号"() -> (w376:string)
        n210 = Format Into String(format string="编号：%s\n参数：%s\n信息：%s" ("格式字符串"), w376, "藻密度" ("输入 2"), w374) -> (resulting string=w373:string)  [unwired: 2 in, 1 out]
        n211 = One Button Dialog(message=w373) -> ()  [unwired: 1 in, 1 out]
        n212 = call "操作日志.vi"("table"="校准记录", "日志信息"=w373) -> ("error out"=w378:errorcluster)  [unwired: 9 in]
      }
      frame "校准结束" {
        n213 = local read "提示"() -> (w400:string)
      }
    }
    "提示" <- w105
  }
